vi "volt vs retardance.vi"(11 "file path (dialog if empty)":path) -> (2 "retardance in degree(known)":dbl[](array[numeric]), 3 "Voltage(unknown)":dbl[](array[numeric]))   [LabVIEW 2014]
uses:
  <vilib>/Utility/file.llb/Read From Spreadsheet File (DBL).vi
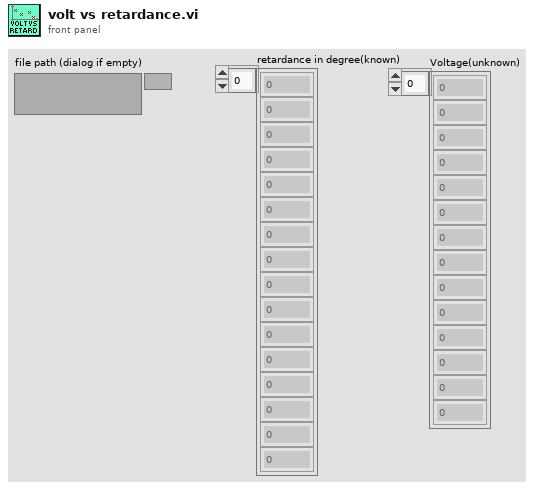
[diagram p1: front panel]
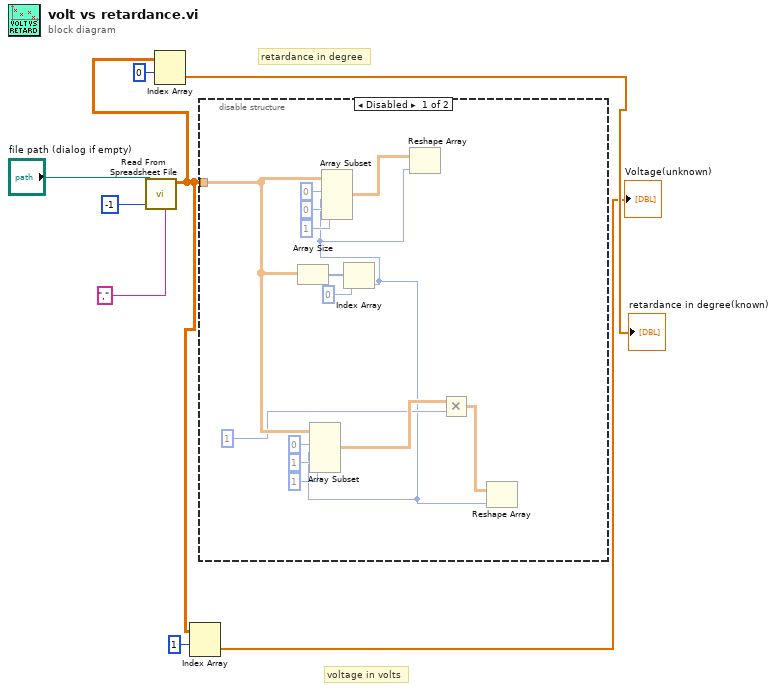
[diagram p0: block diagram]
diagram:
  # "voltage in volts"
  # "retardance in degree"
  n1 = call-poly <vilib>:"Read From Spreadsheet File.vi"("delimiter (\\t)"="," ("delimiter (\\t)"), "number of rows (all:-1)"=-1, "file path (dialog if empty)"="file path (dialog if empty)") -> ("all rows"=w3:dbl[][])  [unwired: 4 in, 4 out]
  n2 = Index Array(array=w3, index (row)=0) -> (element=→"retardance in degree(known)":dbl[])  [unwired: 1 in]
  n3 = Index Array(array=w3, index (row)=1) -> (element=→"Voltage(unknown)":dbl[])  [unwired: 1 in]
  n4 = disable-structure shown="Disabled" {
    disable-tunnel: w3 -> [w14 _]
    frame Disabled {
      n5 = Array Size(array=w14) -> (size(s)=w20:i32[])
      n6 = Index Array(array=w20, index=0) -> (element=w9:i32)
      n7 = Array Subset(array=w14, index (row)=0 ("index"), length (row)=w9, index (col)=1 ("index"), length (col)=1 ("length")) -> (w13:dbl[][])
      n8 = Array Subset(array=w14, index (row)=0 ("index"), length (row)=w9, index (col)=0 ("index"), length (col)=1 ("length")) -> (w11:dbl[][])
      n9 = Reshape Array(w11, w9) -> ()  [unwired: 1 out]
      n10 = Multiply(x=w13, y=1 ("element")) -> (x*y=w10:dbl[][])
      n11 = Reshape Array(w10, w9) -> ()  [unwired: 1 out]
    }
    frame Enabled {
    }
  }
